vi "arduinoTest.vi"() -> ()   [LabVIEW 2021]
uses:
  Program Files/National Instruments/LabVIEW 2021/examples/Instrument IO/Serial/support/Serial - Settings.ctl
  <vilib>/Instr/_visa.llb/VISA Configure Serial Port (Instr).vi
panel:
  in  "stop":bool
  in  "647nm":bool
  in  "553nm":bool
  in  "488nm":bool
  out "error out":errorcluster
  in  "Serial Settings":T1={"baud rate"=9600, "data bits"=8, "parity"=enum."None", "stop bits"=10, "flow control"=0} {"flow control" items=["None"=0, "XON/XOFF"=1, "RTS/CTS"=2, "DTR/DSR"=4]; "stop bits" items=["1.0"=10, "1.5"=15, "2.0"=20]; "data bits" min=5 max=8 step=1; "baud rate" items=["75"=75, "110"=110, "134"=134, "150"=150, "300"=300, "600"=600, "1200"=1200, "1800"=1800, "2400"=2400, "4800"=4800, "7200"=7200, "9600"=9600, "14400"=14400, "19200"=19200, "28800"=28800, "38400"=38400, "56000"=56000, "57600"=57600, "115200"=115200, "128000"=128000, "230400"=230400]}
  in  "VISA resource name":refnum<visa-resource-name>="COM12"
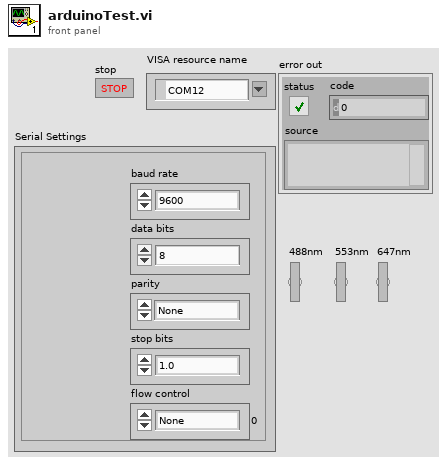
[diagram p1: front panel]
types:
  T1 = typedef "Serial - Settings.ctl" = cluster{"baud rate":u32, "data bits":u16, "parity":enum16{"None", "Odd", "Even", "Mark", "Space"}, "stop bits":u16, "flow control":u16}
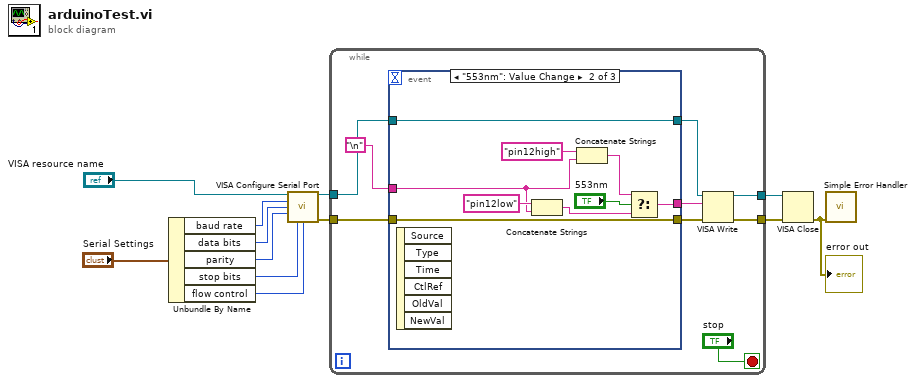
[diagram p0: block diagram]
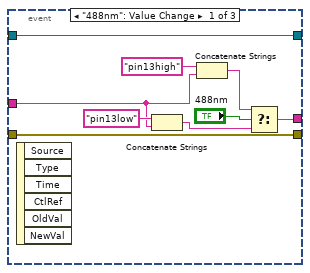
[diagram p2: hidden frame]
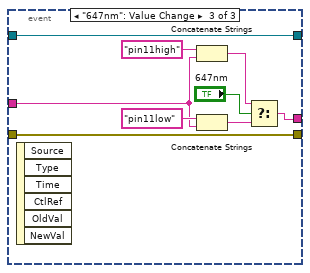
[diagram p3: hidden frame]
diagram:
  n1 = Unbundle By Name("Serial Settings") -> ("baud rate"=w8:u32, "data bits"=w9:u16, "parity"=w10:enum16{"None", "Odd", "Even", "Mark", "Space"}, "stop bits"=w11:u16, "flow control"=w12:u16)
  n2 = call-poly "VISA Configure Serial Port"("VISA resource name"="VISA resource name", "baud rate (9600)"=w8, "data bits (8)"=w9, "parity (0:none)"=w10, "stop bits (10: 1 bit)"=w11, "flow control (0:none)"=w12) -> ("VISA resource name out"=w5:refnum<visa-resource-name>, "error out"=w4:errorcluster)  [unwired: 3 in, 5 out]
  n3 = while {
    tunnel: w5 -> [w19]
    tunnel: [w16] -> w1
    tunnel: w4 -> [w20]
    tunnel: [w15] -> w2
    stop <- "stop" stop-if-true
    n4 = event shown="[1] \"553nm\": Value Change" {
      selector: _ -> [_ _ _]
      dyn-events: _ -> [_ _ _]
      timeout: _ -> [_ _ _]
      tunnel: w20 -> [w23 w31 w40]
      tunnel: "\n" -> [w26 w35 w44]
      tunnel: w19 -> [w24 w33 w42]
      tunnel: [w24 w33 w42] -> w17
      tunnel: [w23 w31 w40] -> w14
      tunnel: [w22 w32 w41] -> w18
      event "488nm": Value Change {
        n5 = event-data() -> ()  [unwired: 1 in, 6 out]
        n6 = Concatenate Strings("pin13low", w26) -> (w30:string)
        n7 = Concatenate Strings("pin13high", w26) -> (w28:string)
        n8 = Select(t=w28, s="488nm", f=w30) -> (s? t:f=w22:string)
      }
      event "553nm": Value Change {
        n9 = event-data() -> ()  [unwired: 1 in, 6 out]
        n10 = Concatenate Strings("pin12low", w35) -> (w39:string)
        n11 = Concatenate Strings("pin12high", w35) -> (w37:string)
        n12 = Select(t=w37, s="553nm", f=w39) -> (s? t:f=w32:string)
      }
      event "647nm": Value Change {
        n13 = event-data() -> ()  [unwired: 1 in, 6 out]
        n14 = Concatenate Strings("pin11high", w44) -> (w46:string)
        n15 = Concatenate Strings("pin11low", w44) -> (w48:string)
        n16 = Select(t=w46, s="647nm", f=w48) -> (s? t:f=w41:string)
      }
    }
    n17 = VISA Write(VISA resource name=w17, write buffer=w18, error in (no error)=w14) -> (VISA resource name out=w16:refnum<visa-resource-name>, error out=w15:errorcluster)  [unwired: 1 out]
  }
  n18 = VISA Close(VISA resource name=w1, error in (no error)=w2) -> (error out=w3:errorcluster)
  "error out" <- w3
  n19 = call <vilib>:"Simple Error Handler.vi"("error in (no error)"=w3) -> ()  [unwired: 1 in, 8 out]
